vi "Read Payload Length.vi"(8 "error in (no error)":errorcluster, 11 "CIFFIFO in":refnum<class "CIFfifo.lvclass">) -> (0 "error out":errorcluster, 2 "Length":u64, 3 "CIFFIFO out":refnum<class "CIFfifo.lvclass">)   [LabVIEW 2021, in "CIFfifo.lvclass"]
uses:
  CIFfifo.lvclass
  CIFfifo.lvclass/CIFfifo.ctl
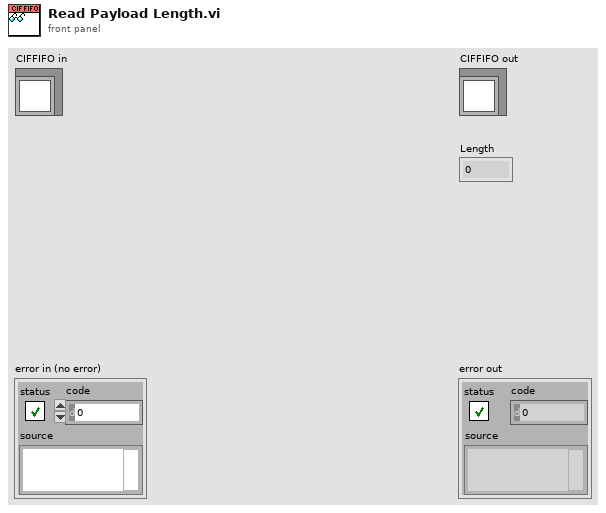
[diagram p1: front panel]
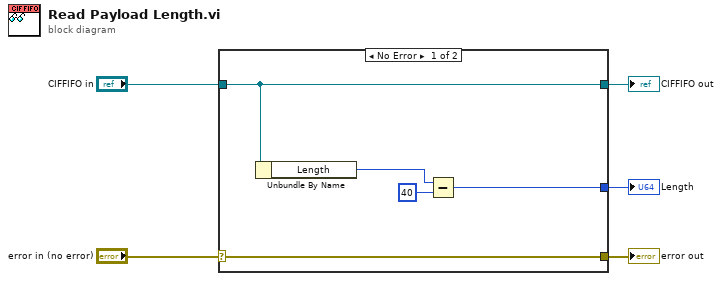
[diagram p0: block diagram]
diagram:
  n1 = case shown="No Error" "error in (no error)" {
    selector: "error in (no error)" -> [w10 w11]
    tunnel: [w10 w11] -> w4
    tunnel: [w9 w12] -> w2
    tunnel: "CIFFIFO in" -> [w9 w12]
    tunnel: [w7 _] -> w1
    frame No Error {
      n2 = Unbundle By Name(w9) -> ("Length"=w8:u64)
      n3 = Subtract(x=w8, y=u64 40) -> (x-y=w7:u64)
    }
    frame Error {
    }
  }
  "error out" <- w4
  "CIFFIFO out" <- w2
  "Length" <- w1
